vi "Element Init.vi"(7 "VolatusAPI":refnum<class "VolatusAPI.lvclass">, 8 "error in (no error)":errorcluster, 10 "JSON":string, 11 "SimpleChart in":refnum<class "SimpleChart.lvclass">) -> (0 "error out":errorcluster, 3 "SimpleChart out":refnum<class "SimpleChart.lvclass">)   [LabVIEW 2020, in "VolatusGUIElements.lvlib" / "SimpleChart.lvclass"]
uses:
  SimpleChart.lvclass
  SimpleChart.lvclass/SimpleChart.ctl
  a5a3055b-817c-4971-bfe2-e27248d2769c.vi
  JSON.ctl
  Volatus/VolatusAPI/VolatusAPI.lvclass
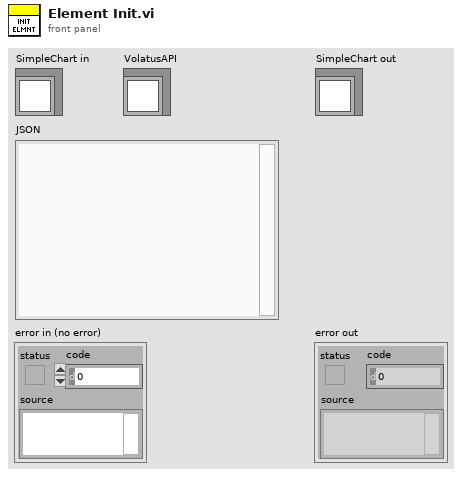
[diagram p1: front panel]
types:
  T1 = typedef "VolatusGUIElements.lvlib/SimpleChart.lvclass/JSON.ctl" = cluster{"Channels":string[]}
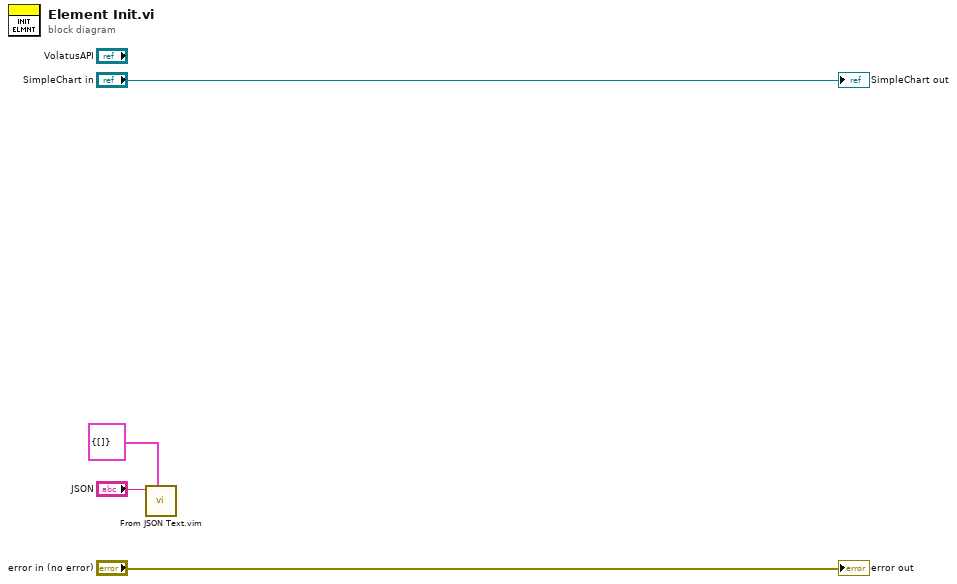
[diagram p0: block diagram]
diagram:
  n1 = call "From JSON Text.vim"("Data Type and Default Value"=T1 {"Channels"=[]} ("JSON"), "JSON"="JSON") -> ()  [unwired: 8 in, 2 out]
  "error out" <- "error in (no error)"
  "SimpleChart out" <- "SimpleChart in"
